vi "Control_Continuous_Send_Loop.vi"(0 "Cont Send":refnum<queue>, 2 "Cont Send Loop Control Command":T1, 11 "Error In":errorcluster) -> (15 "Error Out":errorcluster)   [LabVIEW 2016]
uses:
  type defs/Cont_Send_Loop_Control_Command.ctl
  type defs/Cont_Send_States.ctl
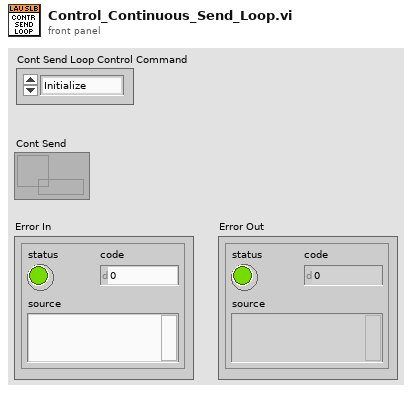
[diagram p1: front panel]
types:
  T1 = typedef "Cont_Send_Loop_Control_Command.ctl" = enum16{"Initialize", "Shutdown"}
  T2 = typedef "Cont_Send_States.ctl" = enum16{"Run", "Shutdown"}
  T3 = typedef "Ref_Cont_Send_Queue.ctl" = refnum<queue>
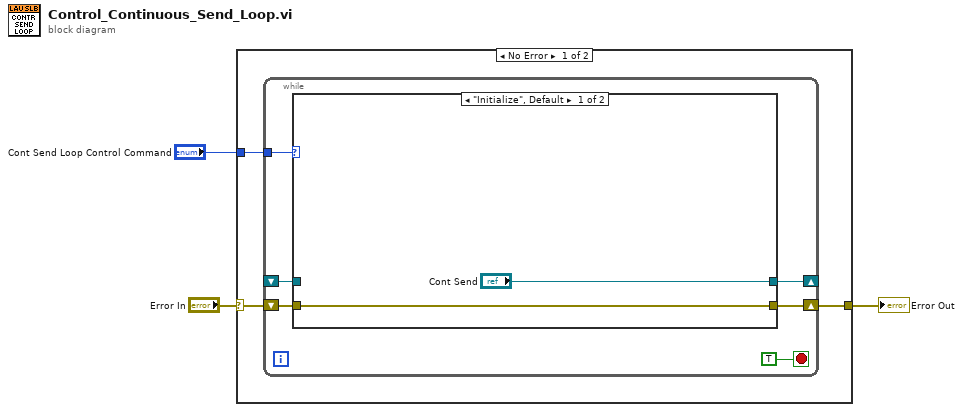
[diagram p0: block diagram]
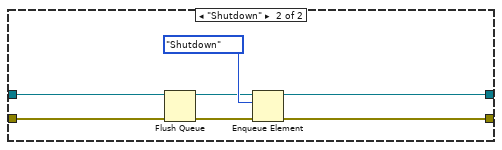
[diagram p2: hidden frame]
diagram:
  n1 = case shown="No Error" "Error In" {
    selector: "Error In" -> [w5 w22]
    tunnel: "Cont Send Loop Control Command" -> [w6 _]
    tunnel: [w4 w22] -> w2
    frame No Error {
      n2 = while {
        tunnel: w6 -> [w12]
        shift-right: [w9] -> w4
        shift-left: w5 -> [w10]
        shift-right: [w8] -> _
        shift-left: _ -> [w7]
        stop <- TRUE stop-if-true
        n3 = case shown="\"Initialize\", Default" w12 {
          tunnel: w10 -> [w14 w21]
          tunnel: [w14 w19] -> w9
          tunnel: ["Cont Send" w15] -> w8
          tunnel: w7 -> [_ w17]
          frame "Initialize", Default {
          }
          frame "Shutdown" {
            n4 = Flush Queue(queue=w17, error in (no error)=w21) -> (queue out=w16:T3, error out=w20:errorcluster)  [unwired: 1 out]
            n5 = Enqueue Element(queue=w16, element=Cont_Send_States."Shutdown", error in (no error)=w20) -> (queue out=w15:T3, error out=w19:errorcluster)  [unwired: 1 in, 1 out]
          }
        }
      }
    }
    frame Error {
    }
  }
  "Error Out" <- w2
